vi "API Folder.vi"() -> (2 "API Folder":path, 3 "API Zip":path)   [LabVIEW 2021]
doc: "Returns the paths for the LabVIEW API folder and the backup zip file."
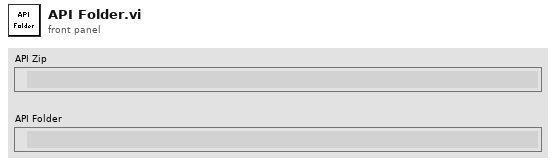
[diagram p1: front panel]
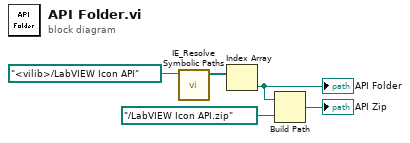
[diagram p0: block diagram]
diagram:
  n1 = call <resource>:"IE_Resolve Symbolic Paths.vi"("symbolic path"=path "<vilib>/LabVIEW Icon API") -> ("resolved paths"=w2:path[])  [unwired: 10 in]
  n2 = Index Array(array=w2) -> (element=w1:path)  [unwired: 1 in]
  "API Folder" <- w1
  n3 = Build Path(base path=w1, name or relative path=path "../LabVIEW Icon API.zip") -> (appended path=→"API Zip":path)
